vi "Byte Buffer.Mapping.Read Typed Array.vi"(0 "Byte Buffer in":refnum<class "Byte Buffer.lvclass">, 1 "data type":T1, 5 "buffer in":dbl[](array[numeric]), 7 "count":i32, 9 "buffer offset":i32, 11 "error in (no error)":errorcluster) -> (4 "Byte Buffer out":refnum<class "Byte Buffer.lvclass">, 6 "buffer out":dbl[](array[numeric]), 10 "new buffer offset":i32, 15 "error out":errorcluster)   [LabVIEW 2016, in "VeriStand Data.lvlib" / "Byte Buffer.lvclass"]
uses:
  Byte Buffer.lvclass
  Typedefs/Typedefs.Data Types.ctl
  Byte Buffer.lvclass/Byte Buffer.ctl
  Byte Buffer.Read (1D Boolean).vi
  Type Conversion/Type Conversion.To Double.Subset (1D Boolean).vi
  Byte Buffer.Read (1D SGL).vi
  Type Conversion/Type Conversion.To Double.Subset (1D SGL).vi
  Byte Buffer.Read (1D DBL).vi
  Byte Buffer.Read (1D I8).vi
  Type Conversion/Type Conversion.To Double.Subset (1D I8).vi
  Byte Buffer.Read (1D I16).vi
  Type Conversion/Type Conversion.To Double.Subset (1D I16).vi
  Byte Buffer.Read (1D I32).vi
  Type Conversion/Type Conversion.To Double.Subset (1D I32).vi
  Byte Buffer.Read (1D I64).vi
  Type Conversion/Type Conversion.To Double.Subset (1D I64).vi
  Byte Buffer.Read (1D U8).vi
  Type Conversion/Type Conversion.To Double.Subset (1D U8).vi
  Byte Buffer.Read (1D U16).vi
  Type Conversion/Type Conversion.To Double.Subset (1D U16).vi
  Byte Buffer.Read (1D U32).vi
  Type Conversion/Type Conversion.To Double.Subset (1D U32).vi
  Byte Buffer.Read (1D U64).vi
  Type Conversion/Type Conversion.To Double.Subset (1D U64).vi
  SubVIs/Sizeof.Scalar.vi
  Type Conversion/Type Conversion.To Double.vi
  Type Conversion/Type Conversion.To Double (1D Boolean).vi
  Type Conversion/Type Conversion.To Double (1D SGL).vi
  Type Conversion/Type Conversion.To Double (1D I8).vi
  Type Conversion/Type Conversion.To Double (1D I16).vi
  Type Conversion/Type Conversion.To Double (1D I32).vi
  Type Conversion/Type Conversion.To Double (1D I64).vi
  Type Conversion/Type Conversion.To Double (1D U8).vi
  Type Conversion/Type Conversion.To Double (1D U16).vi
  Type Conversion/Type Conversion.To Double (1D U32).vi
  Type Conversion/Type Conversion.To Double (1D U64).vi
  VeriStand Data.lvlib
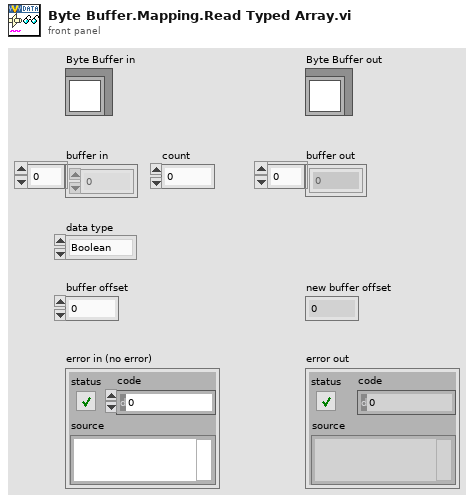
[diagram p1: front panel]
types:
  T1 = typedef "VeriStand Data.lvlib/Typedefs.Data Types.ctl" = enum16{"Boolean", "Single", "Double", "I8", "I16", "I32", "I64", "U8", "U16", "U32", "U64"}
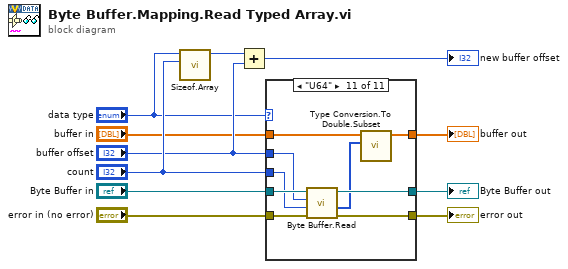
[diagram p0: block diagram]
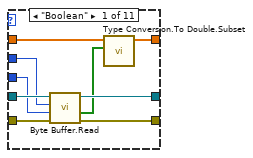
[diagram p2: hidden frame]
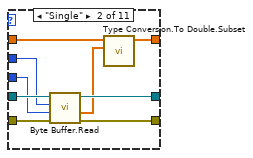
[diagram p3: hidden frame]
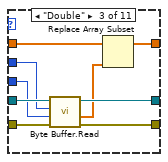
[diagram p4: hidden frame]
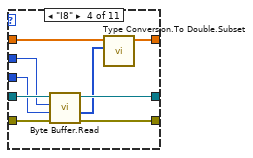
[diagram p5: hidden frame]
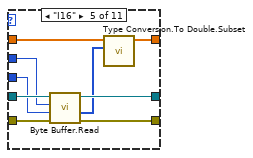
[diagram p6: hidden frame]
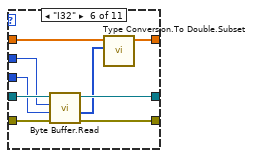
[diagram p7: hidden frame]
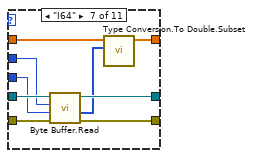
[diagram p8: hidden frame]
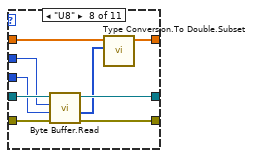
[diagram p9: hidden frame]
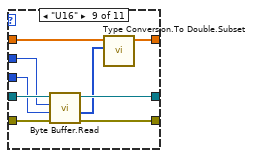
[diagram p10: hidden frame]
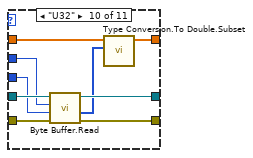
[diagram p11: hidden frame]
diagram:
  n1 = call "Sizeof.Array.vi"("count"="count", "data type"="data type") -> ("size"=w4:i32)  [unwired: 9 in]
  n2 = Add(x=w4, y="buffer offset") -> (x+y=→"new buffer offset":i32)
  n3 = case shown="\"U64\"" "data type" {
    tunnel: "buffer offset" -> [w19 w28 w37 w46 w55 w64 w73 w82 w91 w100 w109]
    tunnel: "Byte Buffer in" -> [w20 w29 w38 w47 w56 w65 w74 w83 w92 w101 w110]
    tunnel: [w13 w22 w33 w40 w49 w58 w67 w76 w85 w94 w103] -> w10
    tunnel: "error in (no error)" -> [w18 w27 w36 w45 w54 w63 w72 w81 w90 w99 w108]
    tunnel: [w16 w25 w34 w43 w52 w61 w70 w79 w88 w97 w106] -> w8
    tunnel: "count" -> [w17 w26 w35 w44 w53 w62 w71 w80 w89 w98 w107]
    tunnel: [w15 w24 w31 w42 w51 w60 w69 w78 w87 w96 w105] -> w6
    tunnel: "buffer in" -> [w14 w23 w32 w41 w50 w59 w68 w77 w86 w95 w104]
    frame "Boolean" {
      n4 = call-poly "Byte Buffer.Read.vi"("error in (no error)"=w18, "count"=w17, "buffer offset"=w19, "Byte Buffer in"=w20) -> ("error out"=w16:errorcluster, "value"=w12:bool[], "Byte Buffer out"=w13:refnum<class "Byte Buffer.lvclass">)  [unwired: 5 in]
      n5 = call-poly "Type Conversion.To Double.Subset.vi"("new values"=w12, "values in"=w14) -> ("values out"=w15:dbl[])  [unwired: 9 in]
    }
    frame "Single" {
      n6 = call-poly "Byte Buffer.Read.vi"("error in (no error)"=w27, "count"=w26, "buffer offset"=w28, "Byte Buffer in"=w29) -> ("error out"=w25:errorcluster, "value"=w21:sgl[], "Byte Buffer out"=w22:refnum<class "Byte Buffer.lvclass">)  [unwired: 5 in]
      n7 = call-poly "Type Conversion.To Double.Subset.vi"("new values"=w21, "values in"=w23) -> ("values out"=w24:dbl[])  [unwired: 9 in]
    }
    frame "Double" {
      n8 = call-poly "Byte Buffer.Read.vi"("error in (no error)"=w36, "count"=w35, "buffer offset"=w37, "Byte Buffer in"=w38) -> ("error out"=w34:errorcluster, "value"=w30:dbl[], "Byte Buffer out"=w33:refnum<class "Byte Buffer.lvclass">)  [unwired: 5 in]
      n9 = Replace Array Subset(array=w32, new element=w30) -> (w31:dbl[])  [unwired: 1 in]
    }
    frame "I8" {
      n10 = call-poly "Byte Buffer.Read.vi"("error in (no error)"=w45, "count"=w44, "buffer offset"=w46, "Byte Buffer in"=w47) -> ("error out"=w43:errorcluster, "value"=w39:i8[], "Byte Buffer out"=w40:refnum<class "Byte Buffer.lvclass">)  [unwired: 5 in]
      n11 = call-poly "Type Conversion.To Double.Subset.vi"("new values"=w39, "values in"=w41) -> ("values out"=w42:dbl[])  [unwired: 9 in]
    }
    frame "I16" {
      n12 = call-poly "Byte Buffer.Read.vi"("error in (no error)"=w54, "count"=w53, "buffer offset"=w55, "Byte Buffer in"=w56) -> ("error out"=w52:errorcluster, "value"=w48:i16[], "Byte Buffer out"=w49:refnum<class "Byte Buffer.lvclass">)  [unwired: 5 in]
      n13 = call-poly "Type Conversion.To Double.Subset.vi"("new values"=w48, "values in"=w50) -> ("values out"=w51:dbl[])  [unwired: 9 in]
    }
    frame "I32" {
      n14 = call-poly "Byte Buffer.Read.vi"("error in (no error)"=w63, "count"=w62, "buffer offset"=w64, "Byte Buffer in"=w65) -> ("error out"=w61:errorcluster, "value"=w57:i32[], "Byte Buffer out"=w58:refnum<class "Byte Buffer.lvclass">)  [unwired: 5 in]
      n15 = call-poly "Type Conversion.To Double.Subset.vi"("new values"=w57, "values in"=w59) -> ("values out"=w60:dbl[])  [unwired: 9 in]
    }
    frame "I64" {
      n16 = call-poly "Byte Buffer.Read.vi"("error in (no error)"=w72, "count"=w71, "buffer offset"=w73, "Byte Buffer in"=w74) -> ("error out"=w70:errorcluster, "value"=w66:i64[], "Byte Buffer out"=w67:refnum<class "Byte Buffer.lvclass">)  [unwired: 5 in]
      n17 = call-poly "Type Conversion.To Double.Subset.vi"("new values"=w66, "values in"=w68) -> ("values out"=w69:dbl[])  [unwired: 9 in]
    }
    frame "U8" {
      n18 = call-poly "Byte Buffer.Read.vi"("error in (no error)"=w81, "count"=w80, "buffer offset"=w82, "Byte Buffer in"=w83) -> ("error out"=w79:errorcluster, "value"=w75:u8[], "Byte Buffer out"=w76:refnum<class "Byte Buffer.lvclass">)  [unwired: 5 in]
      n19 = call-poly "Type Conversion.To Double.Subset.vi"("new values"=w75, "values in"=w77) -> ("values out"=w78:dbl[])  [unwired: 9 in]
    }
    frame "U16" {
      n20 = call-poly "Byte Buffer.Read.vi"("error in (no error)"=w90, "count"=w89, "buffer offset"=w91, "Byte Buffer in"=w92) -> ("error out"=w88:errorcluster, "value"=w84:u16[], "Byte Buffer out"=w85:refnum<class "Byte Buffer.lvclass">)  [unwired: 5 in]
      n21 = call-poly "Type Conversion.To Double.Subset.vi"("new values"=w84, "values in"=w86) -> ("values out"=w87:dbl[])  [unwired: 9 in]
    }
    frame "U32" {
      n22 = call-poly "Byte Buffer.Read.vi"("error in (no error)"=w99, "count"=w98, "buffer offset"=w100, "Byte Buffer in"=w101) -> ("error out"=w97:errorcluster, "value"=w93:u32[], "Byte Buffer out"=w94:refnum<class "Byte Buffer.lvclass">)  [unwired: 5 in]
      n23 = call-poly "Type Conversion.To Double.Subset.vi"("new values"=w93, "values in"=w95) -> ("values out"=w96:dbl[])  [unwired: 9 in]
    }
    frame "U64" {
      n24 = call-poly "Byte Buffer.Read.vi"("error in (no error)"=w108, "count"=w107, "buffer offset"=w109, "Byte Buffer in"=w110) -> ("error out"=w106:errorcluster, "value"=w102:u64[], "Byte Buffer out"=w103:refnum<class "Byte Buffer.lvclass">)  [unwired: 5 in]
      n25 = call-poly "Type Conversion.To Double.Subset.vi"("new values"=w102, "values in"=w104) -> ("values out"=w105:dbl[])  [unwired: 9 in]
    }
  }
  "error out" <- w8
  "Byte Buffer out" <- w10
  "buffer out" <- w6
